vi "to_steps.vi"(8 "Radio Buttons":enum32{"run valve", "bypass valve"}(radio), 11 "Turns":dbl) -> (3 "Steps":i32)   [LabVIEW 2019]
uses:
  global_motor.vi
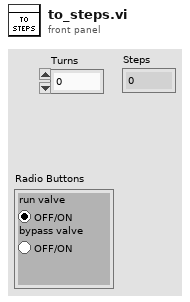
[diagram p1: front panel]
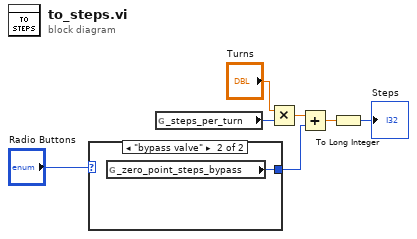
[diagram p0: block diagram]
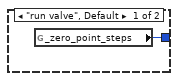
[diagram p2: hidden frame]
diagram:
  n1 = case shown="\"bypass valve\"" "Radio Buttons" {
    tunnel: [w8 w9] -> w1
    frame "run valve", Default {
      n2 = global read "global_motor.vi" "_zero_point_steps"() -> (w8:i32)
    }
    frame "bypass valve" {
      n3 = global read "global_motor.vi" "_zero_point_steps_bypass"() -> (w9:i32)
    }
  }
  n4 = global read "global_motor.vi" "_steps_per_turn"() -> (w3:i32)
  n5 = Multiply(x="Turns", y=w3) -> (x*y=w6:dbl)
  n6 = Add(x=w6, y=w1) -> (x+y=w5:dbl)
  n7 = To Long Integer(number=w5) -> (32bit integer=→"Steps":i32)
